vi "medicaoIXV.vi"() -> ()   [LabVIEW 2012]
uses:
  <vilib>/Utility/file.llb/Write To Spreadsheet File (string).vi
  <vilib>/Utility/file.llb/Write To Spreadsheet File (DBL).vi
  <instrlib>/Agilent 6XXX Series/Agilent 6XXX Series.lvlib
panel:
  out "reset graph":bool=TRUE
  out "array":dbl[][](array[numeric])
  in  "Tab Control":enum32{"Entrada de dados", "Saída de dados"}(tab)
  in  "Área da célula":string
  in  "Tipo da célula":string
  in  "Formato":u16(ring) items=[".txt", ".csv"]
  out "ON/OFF1":bool caption="ON/OFF"
  in  "Pontos":dbl
  in  "Tensão máxima":dbl
  in  "Nome da célula":string
  in  "Local":path
  in  "Delay(ms)":dbl
  in  "Start":bool
  in  "stopProgram":bool caption="Parar Programa"
  out "Imp":dbl
  out "Vmp":dbl
  out "Pmp":dbl
  out "Icc (A)":dbl
  out "Vca (V)":dbl
  in  "Print Screen":bool
  out "IXV":cluster{"Y":dbl[], "Y":dbl[]}[](graph)
  out "output voltage":dbl
  out "Tensao Atual (V)":dbl
  out "Corrente Atual\n(A)":dbl
  out "Ponto Atual":i32
  out "TABELA DE DADOS\nTensão(fonte)     Tensão                  Corrente            Pontos":dbl[][](array[numeric]) caption="all rows" format="%0.3f"
  in  "stop":bool caption="Parar Medição"
  out "ON/OFF2":bool caption="ON/OFF"
  in  "CorrenteGraph":dbl
  in  "error in (no error)":errorcluster
  out "error out":errorcluster
  in  "TensaoGraph":dbl
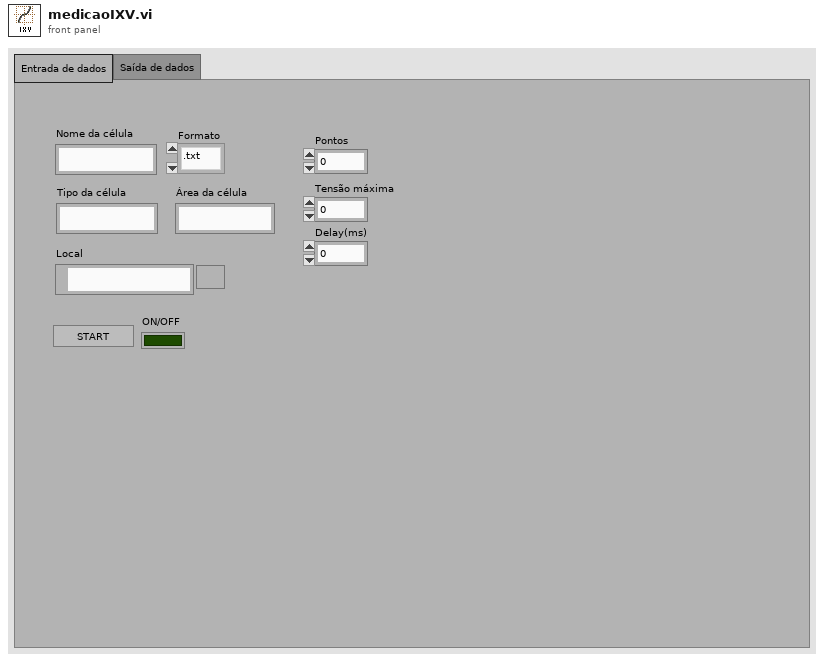
[diagram p1: front panel]
types:
  T1 = typedef "imagedata.ctl" = cluster{"image type":i32, "image depth":i32, "image":u8[], "mask":u8[], "colors":u32[], "Rectangle":cluster{"left":i16, "top":i16, "right":i16, "bottom":i16}}
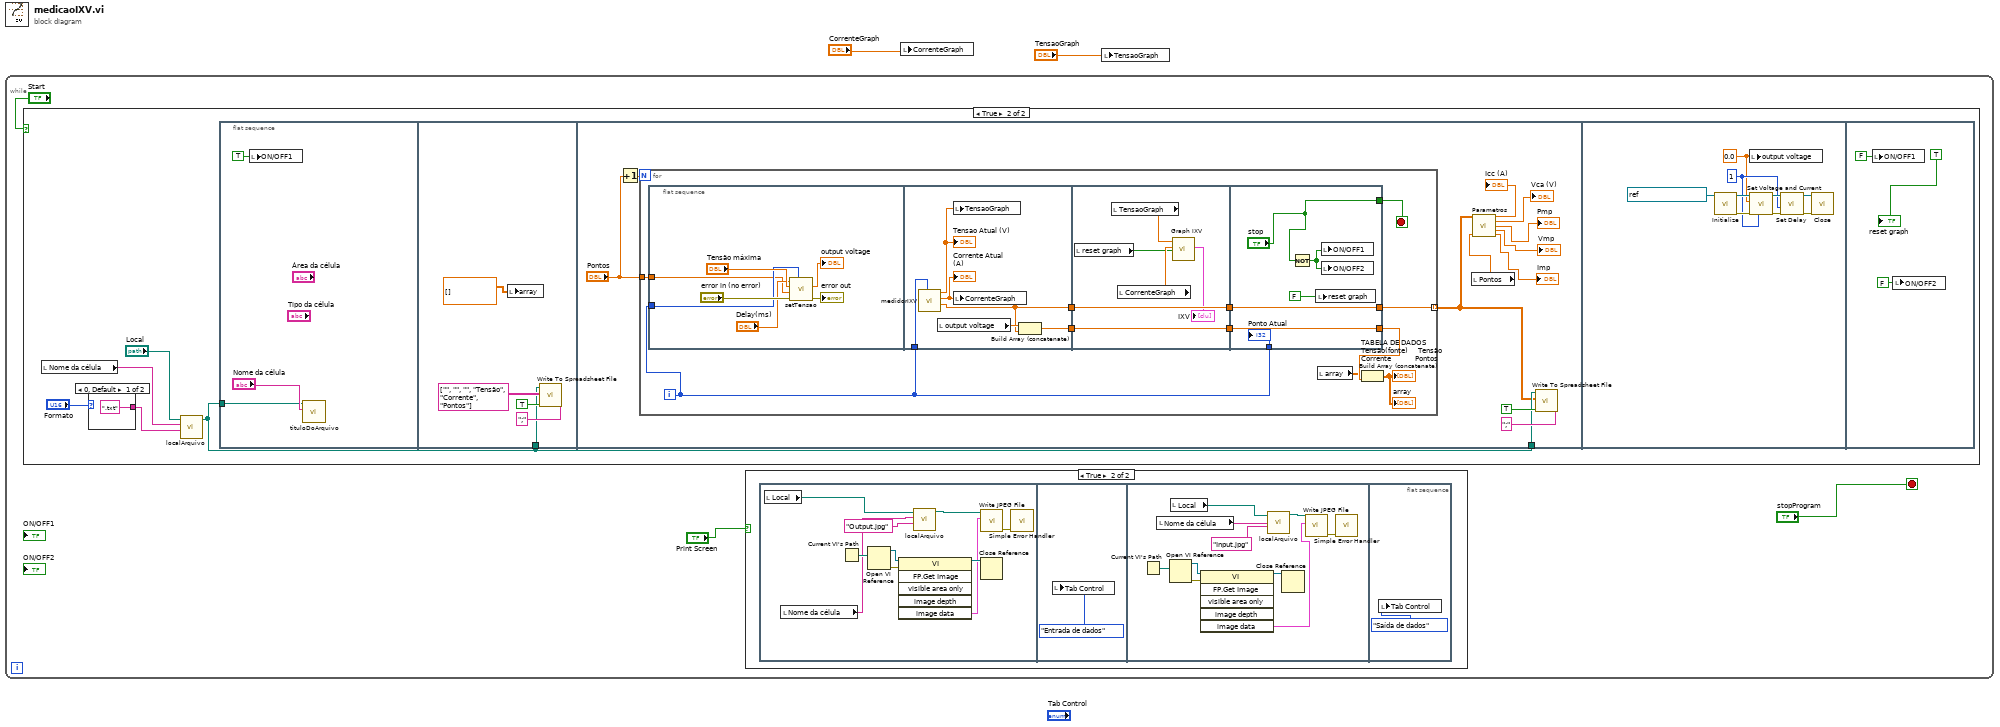
[diagram p0: block diagram]
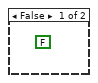
[diagram p3: hidden frame]
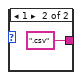
[diagram p4: hidden frame]
diagram:
  n1 = while {
    stop <- "stopProgram" stop-if-true
    n2 = case shown="True" "Start" {
      frame False {
        (unwired) FALSE
      }
      frame True {
        n3 = local read "Nome da célula"() -> (w31:string)
        n4 = case shown="0, Default" "Formato" {
          tunnel: [".txt" ".csv"] -> w28
          frame 0, Default {
          }
          frame 1 {
          }
        }
        n5 = call "localArquivo.vi"("extensão"=w28, "Nome do arquivo"=w31, "Local"="Local") -> ("Path"=w30:path)  [unwired: 8 in]
        n6 = flat-sequence {
          tunnel: w30 -> [w36]
          tunnel: w30 -> [w39]
          tunnel: w30 -> [w52]
          frame #0 {
            n7 = local write "ON/OFF1"(TRUE ("ON/OFF")) -> ()
            n8 = call "tituloDoArquivo.vi"("Nome da célula"="Nome da célula", "file path (dialog if empty)"=w36) -> ()  [unwired: 10 in]
          }
          frame #1 {
            n9 = local write "array"(dbl[][] [] ("array")) -> ()
            n10 = call-poly <vilib>:"Write To Spreadsheet File.vi"("delimiter (\\t)"=";" ("delimiter (\\t)"), "append to file? (new file:F)"=TRUE, "2D data"=string[][] [["", "", ""], ["Tensão", "Corrente", "Pontos"]], "file path (dialog if empty)"=w39) -> ()  [unwired: 4 in, 1 out]
          }
          frame #2 {
            n11 = Increment(x="Pontos") -> (x+1=w51:dbl)
            n12 = for {
              N: w51 -> [_]
              tunnel: [w64] -> w49 mode=indexing
              tunnel: "Pontos" -> [w65]
              i -> [w58]
              stop <- w57 stop-if-true
              n13 = flat-sequence {
                tunnel: w65 -> [w68]
                tunnel: w58 -> [w69]
                tunnel: w58 -> [w78]
                tunnel: [w75] -> w63
                tunnel: [w77] -> w62
                tunnel: [w84] -> w56
                tunnel: [w83] -> w55
                tunnel: w62 -> [w83]
                tunnel: w63 -> [w84]
                tunnel: [w89] -> w61
                tunnel: [w90] -> w64
                tunnel: w56 -> [w90]
                tunnel: w55 -> [w89]
                tunnel: w58 -> [w88]
                tunnel: ["stop"] -> w57
                frame #0 {
                  n14 = call "setTensao.vi"("Ponto"=w69, "error in (no error)"="error in (no error)", "Pontos"=w68, "Tensão máxima"="Tensão máxima", "delay(ms)"="Delay(ms)") -> ("error out"=→"error out":errorcluster, "output voltage"=→"output voltage":dbl)  [unwired: 5 in]
                }
                frame #1 {
                  n15 = call "medidorIXV.vi"("Ponto"=w78) -> ("Array"=w75:dbl[], "Corrente Atual"=w73:dbl, "Tensao Atual"=w74:dbl)  [unwired: 8 in]
                  "Corrente Atual\n(A)" <- w73
                  "Tensao Atual (V)" <- w74
                  n16 = local read "output voltage"() -> (w76:dbl)
                  n17 = local write "TensaoGraph"(w74) -> ()
                  n18 = local write "CorrenteGraph"(w73) -> ()
                  n19 = Build Array (concatenate)(w76, w75) -> (w77:dbl[])
                }
                frame #2 {
                  n20 = local read "reset graph"() -> (w79:bool)
                  n21 = local read "TensaoGraph"() -> (w82:dbl)
                  n22 = local read "CorrenteGraph"() -> (w81:dbl)
                  n23 = call "Graph IXV"("Reset"=w79, "Y Input"=w81, "X Input"=w82) -> ("XY Graph"=→"IXV":cluster{"Y":dbl[], "Y":dbl[]}[])  [unwired: 2 in, 6 out]
                }
                frame #3 {
                  n24 = Not(x="stop") -> (.not. x?=w86:bool)
                  n25 = local write "reset graph"(FALSE) -> ()
                  n26 = local write "ON/OFF1"(w86) -> ()
                  n27 = local write "ON/OFF2"(w86) -> ()
                  "Ponto Atual" <- w88
                }
              }
              n28 = local read "array"() -> (w60:dbl[][])
              n29 = Build Array (concatenate)(w60, w61) -> (→"TABELA DE DADOS\nTensão(fonte)     Tensão                  Corrente            Pontos" →"array":dbl[][])
            }
            n30 = local read "Pontos"() -> (w48:dbl)
            n31 = call "Parametros.vi"("VetorDeDados"=w49, "pontos"=w48) -> ("Icc"=→"Icc (A)":dbl, "Vca"=→"Vca (V)":dbl, "Pmp"=→"Pmp":dbl, "Vmp"=→"Vmp":dbl, "Imp"=→"Imp":dbl)  [unwired: 9 in]
            n32 = call-poly <vilib>:"Write To Spreadsheet File.vi"("delimiter (\\t)"=";" ("delimiter (\\t)"), "append to file? (new file:F)"=TRUE, "2D data"=w49, "file path (dialog if empty)"=w52) -> ()  [unwired: 4 in, 1 out]
          }
          frame #3 {
            w91 = 0.0 ("voltage (0 V)")
            w94 = u8 1 ("channel (1)")
            n33 = call <instrlib>:"Initialize.vi"("VISA resource name"=refnum<visa-resource-name> "GPIB0::5::INSTR") -> ("error out"=w96:errorcluster, "VISA resource name out"=w95:refnum<visa-resource-name>)  [unwired: 9 in]
            n34 = local write "output voltage"(w91) -> ()
            n35 = call <instrlib>:"Set Voltage and Current.vi"("channel (1)"=w94, "error in (no error)"=w96, "voltage (0 V)"=w91, "VISA resource name"=w95) -> ("error out"=w97:errorcluster, "VISA resource name out"=w98:refnum<visa-resource-name>)  [unwired: 6 in]
            n36 = call <instrlib>:"Set Delay.vi"("error in (no error)"=w97, "channel (1)"=w94, "VISA resource name"=w98) -> ("error out"=w92:errorcluster, "VISA resource name out"=w93:refnum<visa-resource-name>)  [unwired: 7 in]
            n37 = call <instrlib>:"Close.vi"("error in (no error)"=w92, "VISA resource name"=w93) -> ()  [unwired: 9 in, 1 out]
          }
          frame #4 {
            n38 = local write "ON/OFF1"(FALSE) -> ()
            n39 = local write "ON/OFF2"(FALSE ("ON/OFF")) -> ()
            "reset graph" <- TRUE
          }
        }
      }
    }
    n40 = case shown="True" "Print Screen" {
      frame False {
      }
      frame True {
        n41 = flat-sequence {
          frame #0 {
            n42 = local read "Local"() -> (w7:path)
            n43 = local read "Nome da célula"() -> (w8:string)
            n44 = Current VI's Path() -> (path=w13:path)
            n45 = Open VI Reference(vi path=w13) -> (vi reference=w14:refnum<vi>, error out=w15:errorcluster)  [unwired: 5 in]
            n46 = invoke class="VI" method="FP.Get Image"(reference=w14, error in=w15) -> (reference out=w12:refnum<vi>, "image data"=w11:T1)  [unwired: 4 in, 4 out]
            n47 = call "localArquivo.vi"("extensão"="Output.jpg", "Nome do arquivo"=w8, "Local"=w7) -> ("Path"=w6:path)  [unwired: 8 in]
            n48 = call <vilib>:"Write JPEG File.vi"("image data"=w11, "path to JPEG file"=w6) -> ("error out"=w10:errorcluster)  [unwired: 8 in, 1 out]
            n49 = Close Reference(reference=w12) -> ()  [unwired: 1 in, 1 out]
            n50 = call <vilib>:"Simple Error Handler.vi"("error in (no error)"=w10) -> ()  [unwired: 4 in, 5 out]
          }
          frame #1 {
            n51 = local write "Tab Control"(enum32{"Entrada de dados", "Saída de dados"}."Entrada de dados" ("Tab Control")) -> ()
          }
          frame #2 {
            n52 = Current VI's Path() -> (path=w25:path)
            n53 = local read "Nome da célula"() -> (w19:string)
            n54 = Open VI Reference(vi path=w25) -> (vi reference=w24:refnum<vi>, error out=w23:errorcluster)  [unwired: 5 in]
            n55 = local read "Local"() -> (w18:path)
            n56 = invoke class="VI" method="FP.Get Image"(reference=w24, error in=w23) -> (reference out=w26:refnum<vi>, "image data"=w21:T1)  [unwired: 4 in, 4 out]
            n57 = call "localArquivo.vi"("extensão"="Input.jpg", "Nome do arquivo"=w19, "Local"=w18) -> ("Path"=w17:path)  [unwired: 8 in]
            n58 = Close Reference(reference=w26) -> ()  [unwired: 1 in, 1 out]
            n59 = call <vilib>:"Write JPEG File.vi"("image data"=w21, "path to JPEG file"=w17) -> ("error out"=w22:errorcluster)  [unwired: 8 in, 1 out]
            n60 = call <vilib>:"Simple Error Handler.vi"("error in (no error)"=w22) -> ()  [unwired: 4 in, 5 out]
          }
          frame #3 {
            n61 = local write "Tab Control"(enum32{"Entrada de dados", "Saída de dados"}."Saída de dados" ("Tab Control")) -> ()
          }
        }
      }
    }
  }
  n62 = local write "CorrenteGraph"("CorrenteGraph") -> ()
  n63 = local write "TensaoGraph"("TensaoGraph") -> ()
